vi "UnloadAction.vi"(8 "error in (no error)":errorcluster caption="entrée d'erreur (pas d'erreur)", 11 "DAQ6363 In":refnum<class "DAQ6363.lvclass"> caption="DNL_LabVIEW Object in") -> (0 "error out":errorcluster caption="sortie d'erreur", 3 "DAQ6363 Out":refnum<class "DAQ6363.lvclass"> caption="DNL_LabVIEW Object out")   [LabVIEW 2019, in "DAQ6363.lvclass"]
uses:
  DAQ6363.lvclass
  C:/Programmes Labview/LabscanV1A/DevicesClass/BaseDevice/BaseDevice.lvclass
  BaseDevice/BaseDevice.lvclass
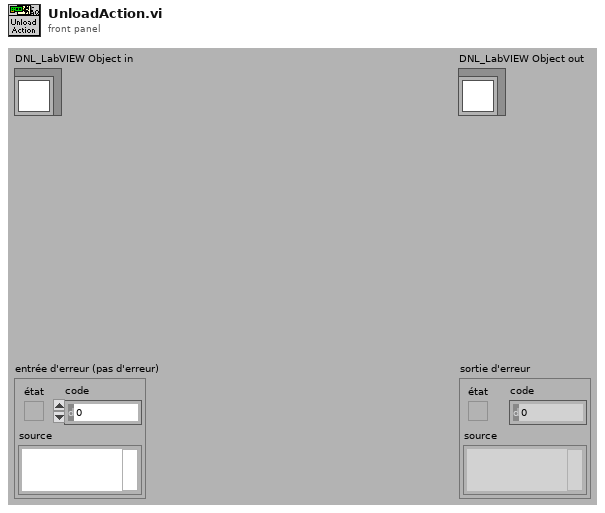
[diagram p1: front panel]
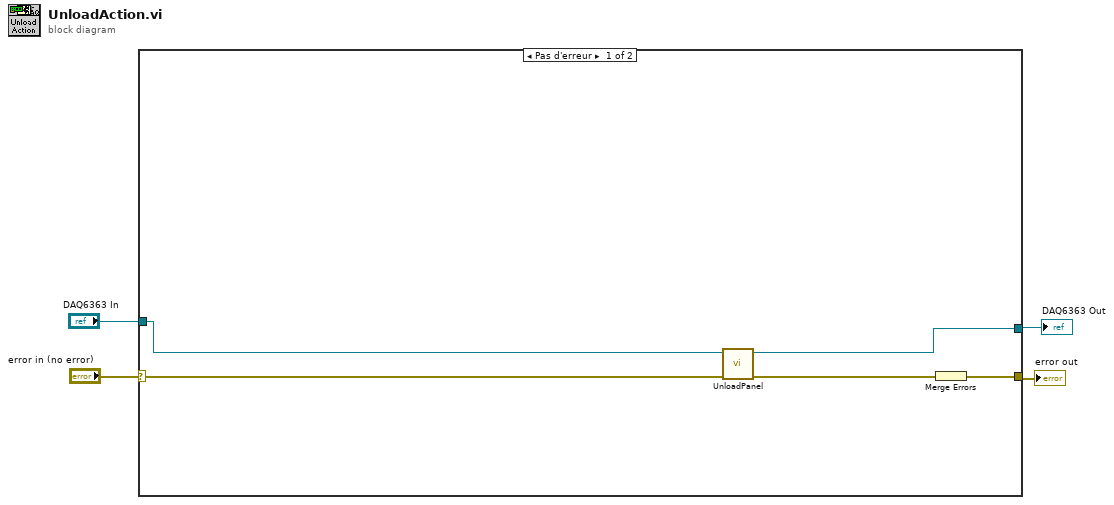
[diagram p0: block diagram]
diagram:
  n1 = case shown="Pas d'erreur" "error in (no error)" {
    selector: "error in (no error)" -> [w7 w10]
    tunnel: [w6 w10] -> w3
    tunnel: [w8 w11] -> w2
    tunnel: "DAQ6363 In" -> [w5 w11]
    frame No Error {
      n2 = call "UnloadPanel.vi"("error in (no error)"=w7, "Device en entrée"=w5) -> ("error out"=w9:errorcluster, "Device en sortie"=w8:refnum<class "DAQ6363.lvclass">)  [unwired: 8 in]
      n3 = Merge Errors(w9) -> (w6:errorcluster)
    }
    frame Error {
    }
  }
  "error out" <- w3
  "DAQ6363 Out" <- w2
